vi "Date2MonthDay.vi"(8 "Error In":errorcluster) -> (0 "Error Out":errorcluster, 3 "MonthDay":string)   [LabVIEW 2014]
doc: "Converts Date String from Get Date/Time \nVI into a String with only the month and\nday."
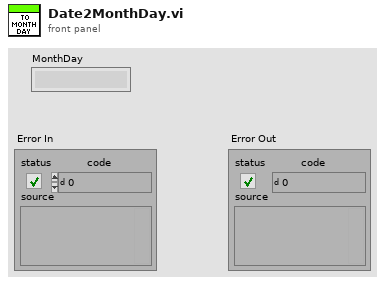
[diagram p1: front panel]
types:
  T1 = enum16{"Jan", "Feb", "Mar", "Apr", "May", "June", "July", "Aug", "Sep", "Oct", "Nov", "Dec"}[]
  T2 = enum16{"Jan", "Feb", "Mar", "Apr", "May", "June", "July", "Aug", "Sep", "Oct", "Nov", "Dec"}
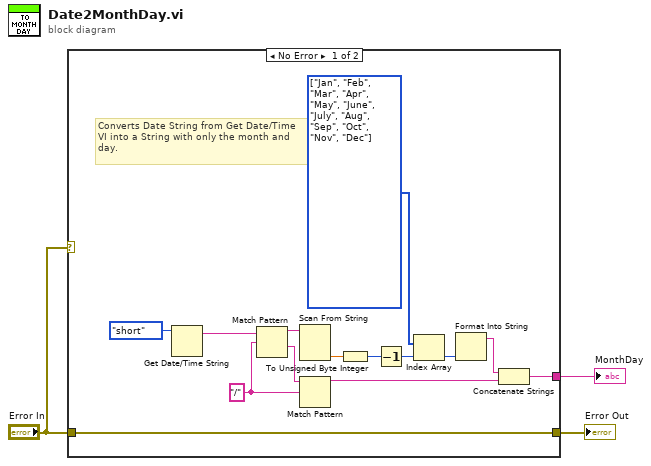
[diagram p0: block diagram]
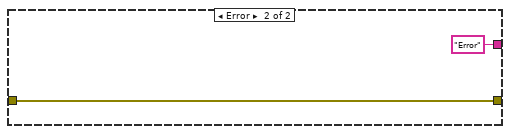
[diagram p2: hidden frame]
diagram:
  n1 = case shown="No Error" "Error In" {
    tunnel: [w17 "Error"] -> w3
    tunnel: [w4 w19] -> w2
    tunnel: "Error In" -> [w4 w19]
    frame No Error {
      w12 = T1 [enum."Jan", enum."Feb", enum."Mar", enum."Apr", enum."May", enum."June", enum."July", enum."Aug", enum."Sep", enum."Oct", enum."Nov", enum."Dec"] items=["Jan", "Feb", "Mar", "Apr", "May", "June", "July", "Aug", "Sep", "Oct", "Nov", "Dec"]
      w8 = "/" ("regular expression")
      # "Converts Date String from Get Date/Time \nVI into a String with only the month and\nday."
      n2 = Get Date/Time String(date format (0)=enum16{"short", "long", "abbreviated"}."short") -> (date string=w6:string)  [unwired: 2 in, 1 out]
      n3 = Match Pattern(string=w6, regular expression=w8) -> (before substring=w9:string, after substring=w7:string)  [unwired: 1 in, 2 out]
      n4 = Scan From String(input string=w9) -> (output 1=w10:dbl)  [unwired: 4 in, 3 out]
      n5 = Match Pattern(string=w7, regular expression=w8) -> (before substring=w16:string)  [unwired: 1 in, 3 out]
      n6 = To Unsigned Byte Integer(number=w10) -> (unsigned 8bit integer=w11:u8)
      n7 = Decrement(x=w11) -> (x-1=w13:u8)
      n8 = Index Array(array=w12, index=w13) -> (element=w14:T2)
      n9 = Format Into String(w14) -> (resulting string=w15:string)  [unwired: 3 in, 1 out]
      n10 = Concatenate Strings(w15, w16) -> (w17:string)
    }
    frame Error {
    }
  }
  "MonthDay" <- w3
  "Error Out" <- w2
